vi "Industrial Parameters.vi"(8 "error in (no error)":errorcluster, 11 "Node Ptr":T1 format="%.0x") -> (0 "error out":errorcluster)   [LabVIEW 2013, in "Control Addon System Explorer.lvlib"]
uses:
  Control Addon System Explorer.lvlib
  <vilib>/NI Veristand/Custom Device API/Custom Device Item Ref.ctl
  Shared/Types/Action.ctl
  Shared/Constants.vi
  <vilib>/NI Veristand/Custom Device API/NI VeriStand - Get Item Property.vi
  <vilib>/NI Veristand/Custom Device API/Get Item Property (Boolean).vi
  <vilib>/NI Veristand/Custom Device API/Get Item Property (Double).vi
  <vilib>/NI Veristand/Custom Device API/NI VeriStand - Set Item Property.vi
  <vilib>/NI Veristand/Custom Device API/Set Item Property (Boolean).vi
  <vilib>/NI Veristand/Custom Device API/Set Item Property (Double).vi
  <vilib>/NI Veristand/Custom Device API/Custom Device API.lvlib
  Shared/Control Addon Shared.lvlib
panel:
  in  "Minimum Switching Duration":dbl caption="Minimum Switching Duration (secs)"
  in  "Setpoint Hysteresis":dbl caption="Setpoint Hysteresis (EU)"
  in  "Enable Hysteresis":bool
  in  "Enable Switching Filter":bool
  in  "Header 2":cluster{"Section Name":string}={"Section Name"="Output Signal Filtering Settings"}
  in  "SHDocVw.IWebBrowser":refnum<k7>(container)
  in  "Header":cluster{"Section Name":string}={"Section Name"="Custom Device Item Settings"}
  in  "Description":string
  out "Name":string
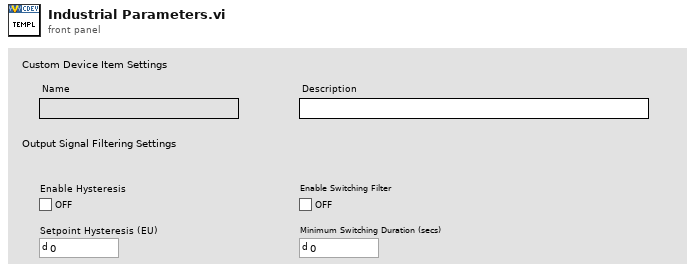
[diagram p1: front panel]
types:
  T1 = typedef "Custom Device API.lvlib/Custom Device Item Ref.ctl" = u64
  T2 = typedef "Control Addon Shared.lvlib/Action.ctl" = enum16{"Get", "Set"}
  T3 = typedef "Control Addon Shared.lvlib/Industrial Parameters.ctl" = cluster{"Enable Hysteresis":bool, "Hysteresis":dbl, "Enable Filter":bool, "Minimum Switching":dbl}
  T4 = typedef "Custom Device API.lvlib/Custom Device Item Info.ctl" = cluster{"Name":string, "Is Channel":bool, "GUID":string, "Is Waveform":bool}
  T5 = typedef "Custom Device API.lvlib/Custom Device Commands.ctl" = enum16{"Default", "Item renamed", "Shutdown", "Dynamic button pressed"}
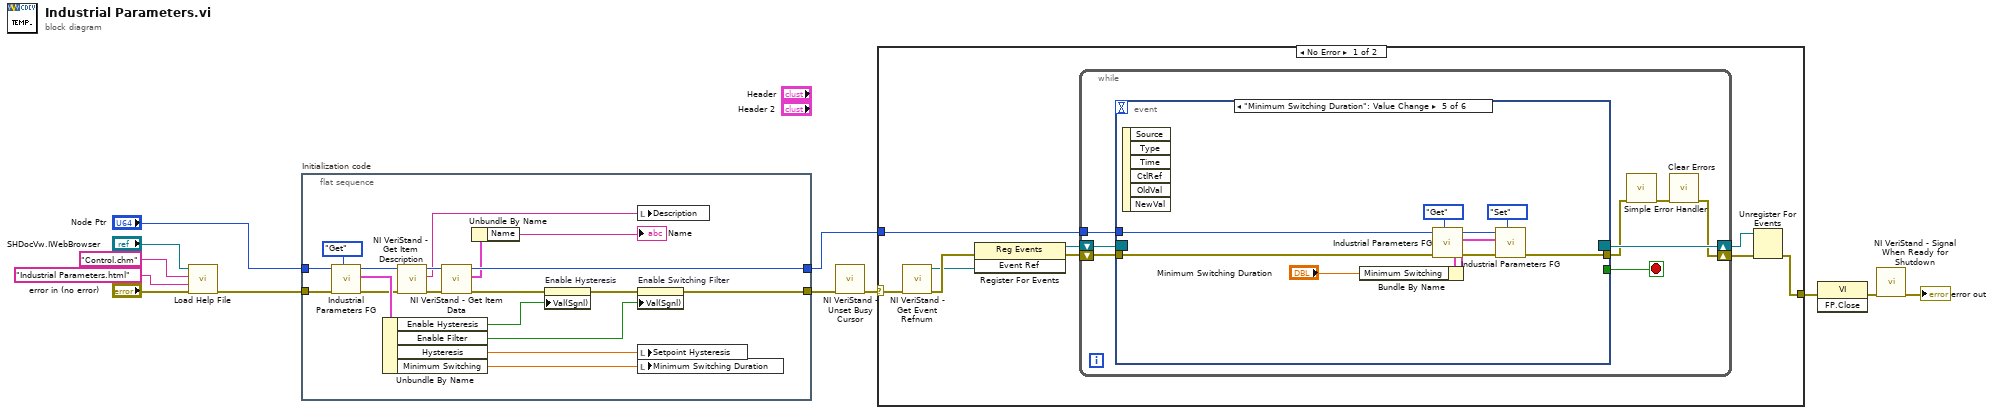
[diagram p0: block diagram]
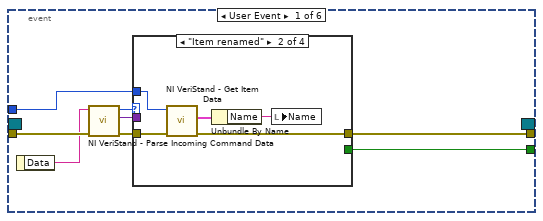
[diagram p2: hidden frame]
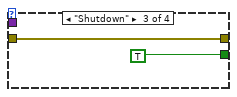
[diagram p4: hidden frame]
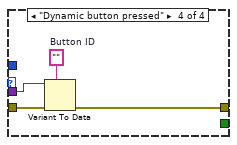
[diagram p5: hidden frame]
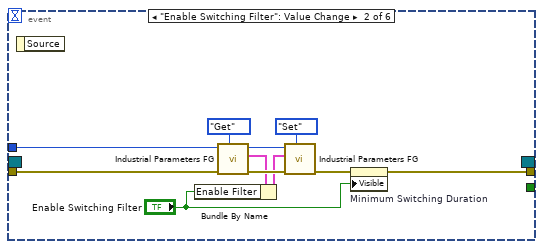
[diagram p6: hidden frame]
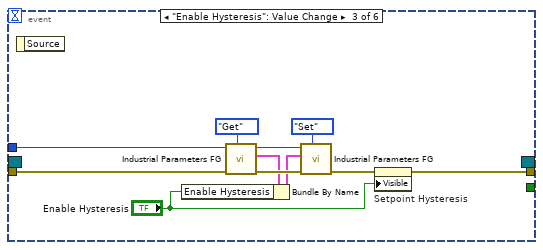
[diagram p7: hidden frame]
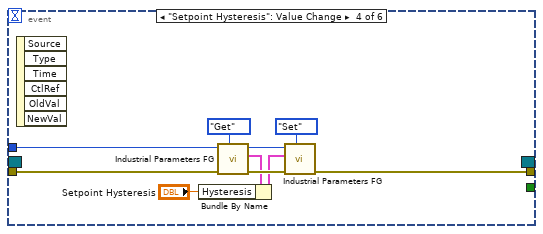
[diagram p8: hidden frame]
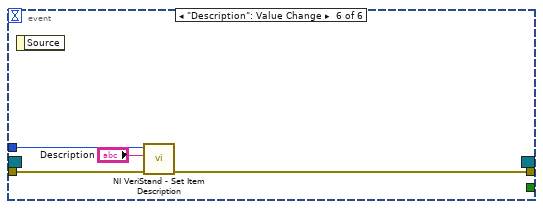
[diagram p9: hidden frame]
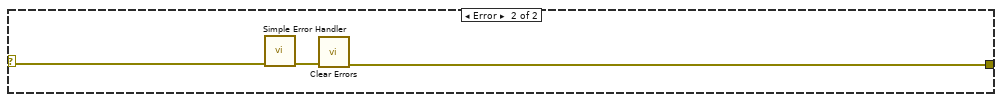
[diagram p10: hidden frame]
diagram:
  n1 = call "Load Help File.vi"("error in (no error)"="error in (no error)", "HTML File"="Industrial Parameters.html", "Main CHM File"="Control.chm", "SHDocVw.IWebBrowser2"="SHDocVw.IWebBrowser") -> ("error out"=w2:errorcluster)  [unwired: 7 in]
  n2 = flat-sequence "Initialization code" {
    tunnel: w2 -> [w25]
    tunnel: "Node Ptr" -> [w24]
    tunnel: [w17] -> w9
    tunnel: [w31] -> w7
    frame #0 {
      n3 = call "Industrial Parameters FG.vi"("Action"=Action."Get", "error in (no error)"=w25, "Node Ptr"=w24) -> ("error out"=w21:errorcluster, "Parameters"=w22:T3, "Item Ref out"=w20:T1)  [unwired: 6 in]
      n4 = Unbundle By Name(w22) -> ("Enable Hysteresis"=w16:bool, "Enable Filter"=w15:bool, "Hysteresis"=w14:dbl, "Minimum Switching"=w13:dbl)
      n5 = call <vilib>:"NI VeriStand - Get Item Description.vi"("error in (no error)"=w21, "Item Ref in"=w20) -> ("error out"=w28:errorcluster, "Description"=w29:string, "Item Ref out"=w30:T1)  [unwired: 7 out]
      n6 = call <vilib>:"NI VeriStand - Get Item Data.vi"("error in (no error)"=w28, "Item Ref in"=w30) -> ("error out"=w18:errorcluster, "Item Info"=w27:T4, "Item Ref out"=w31:T1)  [unwired: 7 out]
      n7 = Unbundle By Name(w27) -> ("Name"=→"Name":string)
      n8 = property on="Enable Hysteresis" class="Bool (strict)"(error in=w18, "Val(Sgnl)"=w16) -> (error out=w19:errorcluster)  [unwired: 1 in, 1 out]
      n9 = local write "Description"(w29) -> ()
      n10 = property on="Enable Switching Filter" class="Bool (strict)"(error in=w19, "Val(Sgnl)"=w15) -> (error out=w17:errorcluster)  [unwired: 1 in, 1 out]
      n11 = local write "Setpoint Hysteresis"(w14) -> ()
      n12 = local write "Minimum Switching Duration"(w13) -> ()
    }
  }
  n13 = call <vilib>:"NI VeriStand - Unset Busy Cursor.vi"("error in (no error)"=w9) -> ("error out"=w8:errorcluster)  [unwired: 10 out]
  n14 = case shown="No Error" w8 {
    selector: w8 -> [w32 w117]
    tunnel: [w37 w115] -> w12
    tunnel: w7 -> [w33 _]
    frame No Error {
      n15 = call <vilib>:"NI VeriStand - Get Event Refnum.vi"("error in (no error)"=w32) -> ("error out"=w40:errorcluster, "Event Ref"=w36:refnum<user-event>)  [unwired: 9 out]
      n16 = register-events(error in=w40, w36) -> (reference out=w34:refnum<event-registration>, error out=w35:errorcluster)  [unwired: 1 in]
      n17 = while {
        tunnel: w33 -> [w44]
        shift-right: [w41] -> w38
        shift-left: w35 -> [w47]
        shift-right: [w48] -> w39
        shift-left: w34 -> [w46]
        stop <- w45 stop-if-true
        n18 = event shown="[4] \"Minimum Switching Duration\": Value Change" {
          selector: w46 -> [_ _ _ _ _ _]
          dyn-events: [_ _ _ _ _ _] -> w48
          timeout: _ -> [_ _ _ _ _ _]
          tunnel: w47 -> [w56 w77 w88 w99 w109 w113]
          tunnel: [w52 _ _ _ _ _] -> w45
          tunnel: [w51 w79 w90 w91 w102 w112] -> w43
          tunnel: w44 -> [w50 w76 w87 w98 w108 w114]
          event User Event {
            n19 = event-data() -> ("Data"=w55:string)  [unwired: 1 out]
            n20 = call <vilib>:"NI VeriStand - Parse Incoming Command Data.vi"("error in (no error)"=w56, "Incoming data"=w55) -> ("error out"=w54:errorcluster, "Outgoing data"=w49:variant, "Action"=w53:T5)  [unwired: 7 out]
            n21 = case shown="\"Item renamed\"" w53 {
              tunnel: w54 -> [w57 w62 w63 w68]
              tunnel: [_ _ TRUE _] -> w52
              tunnel: [w57 w59 w63 w65] -> w51
              tunnel: w50 -> [_ w61 _ _]
              tunnel: w49 -> [_ _ _ w67]
              frame "Default", Default {
              }
              frame "Item renamed" {
                n22 = call <vilib>:"NI VeriStand - Get Item Data.vi"("error in (no error)"=w62, "Item Ref in"=w61) -> ("error out"=w59:errorcluster, "Item Info"=w60:T4)  [unwired: 8 out]
                n23 = Unbundle By Name(w60) -> ("Name"=w58:string)
                n24 = local write "Name"(w58) -> ()
              }
              frame "Shutdown" {
              }
              frame "Dynamic button pressed" {
                w66 = ""  # Button ID
                n25 = Variant To Data(error in=w68, type=w66, Variant=w67) -> (error out=w65:errorcluster)  [unwired: 1 out]
              }
            }
          }
          event "Enable Switching Filter": Value Change {
            n26 = event-data() -> ()  [unwired: 2 out]
            n27 = call "Industrial Parameters FG.vi"("Action"=Action."Get", "error in (no error)"=w77, "Node Ptr"=w76) -> ("error out"=w74:errorcluster, "Parameters"=w71:T3, "Item Ref out"=w72:T1)  [unwired: 6 in]
            n28 = Bundle By Name(cluster=w71, "Enable Filter"="Enable Switching Filter") -> (w70:T3)
            n29 = call "Industrial Parameters FG.vi"("Action"=Action."Set", "error in (no error)"=w74, "Parameters"=w70, "Node Ptr"=w72) -> ("error out"=w73:errorcluster)  [unwired: 5 in, 2 out]
            n30 = property on="Minimum Switching Duration" class="DigNum (strict)"(error in=w73, "Visible"="Enable Switching Filter") -> (error out=w79:errorcluster)  [unwired: 1 in, 1 out]
          }
          event "Enable Hysteresis": Value Change {
            n31 = event-data() -> ()  [unwired: 2 out]
            n32 = call "Industrial Parameters FG.vi"("Action"=Action."Get", "error in (no error)"=w88, "Node Ptr"=w87) -> ("error out"=w85:errorcluster, "Parameters"=w82:T3, "Item Ref out"=w83:T1)  [unwired: 6 in]
            n33 = Bundle By Name(cluster=w82, "Enable Hysteresis"="Enable Hysteresis") -> (w81:T3)
            n34 = call "Industrial Parameters FG.vi"("Action"=Action."Set", "error in (no error)"=w85, "Parameters"=w81, "Node Ptr"=w83) -> ("error out"=w84:errorcluster)  [unwired: 5 in, 2 out]
            n35 = property on="Setpoint Hysteresis" class="DigNum (strict)"(error in=w84, "Visible"="Enable Hysteresis") -> (error out=w90:errorcluster)  [unwired: 1 in, 1 out]
          }
          event "Setpoint Hysteresis": Value Change {
            n36 = event-data() -> ()  [unwired: 7 out]
            n37 = call "Industrial Parameters FG.vi"("Action"=Action."Get", "error in (no error)"=w99, "Node Ptr"=w98) -> ("error out"=w96:errorcluster, "Parameters"=w94:T3, "Item Ref out"=w95:T1)  [unwired: 6 in]
            n38 = Bundle By Name(cluster=w94, "Hysteresis"="Setpoint Hysteresis") -> (w93:T3)
            n39 = call "Industrial Parameters FG.vi"("Action"=Action."Set", "error in (no error)"=w96, "Parameters"=w93, "Node Ptr"=w95) -> ("error out"=w91:errorcluster)  [unwired: 5 in, 2 out]
          }
          event "Minimum Switching Duration": Value Change {
            n40 = event-data() -> ()  [unwired: 7 out]
            n41 = call "Industrial Parameters FG.vi"("Action"=Action."Get", "error in (no error)"=w109, "Node Ptr"=w108) -> ("error out"=w106:errorcluster, "Parameters"=w104:T3, "Item Ref out"=w105:T1)  [unwired: 6 in]
            n42 = Bundle By Name(cluster=w104, "Minimum Switching"="Minimum Switching Duration") -> (w103:T3)
            n43 = call "Industrial Parameters FG.vi"("Action"=Action."Set", "error in (no error)"=w106, "Parameters"=w103, "Node Ptr"=w105) -> ("error out"=w102:errorcluster)  [unwired: 5 in, 2 out]
          }
          event "Description": Value Change {
            n44 = event-data() -> ()  [unwired: 2 out]
            n45 = call <vilib>:"NI VeriStand - Set Item Description.vi"("error in (no error)"=w113, "Description"="Description", "Item Ref in"=w114) -> ("error out"=w112:errorcluster)  [unwired: 8 out]
          }
        }
        n46 = call <vilib>:"Simple Error Handler.vi"("error in (no error)"=w43) -> ("error out"=w42:errorcluster)  [unwired: 1 in, 7 out]
        n47 = call <vilib>:"Clear Errors.vi"("error in (no error)"=w42) -> ("error out"=w41:errorcluster)  [unwired: 6 out]
      }
      n48 = Unregister For Events(event registration refnum=w39, error in=w38) -> (error out=w37:errorcluster)
    }
    frame Error {
      n49 = call <vilib>:"Simple Error Handler.vi"("error in (no error)"=w117) -> ("error out"=w116:errorcluster)  [unwired: 1 in, 7 out]
      n50 = call <vilib>:"Clear Errors.vi"("error in (no error)"=w116) -> ("error out"=w115:errorcluster)  [unwired: 6 out]
    }
  }
  n51 = invoke class="VI" method="FP.Close"(error in=w12) -> (error out=w11:errorcluster)  [unwired: 2 in, 2 out]
  n52 = call <vilib>:"NI VeriStand - Signal When Ready for Shutdown.vi"("error in (no error)"=w11) -> ("error out"=→"error out":errorcluster)  [unwired: 10 out]
